vi "Teleop.vi"(10 "Match Info":T3={"Autonomous Elapsed Seconds"=0.0, "TeleOp Elapsed Seconds"=0.0, "Disabled Elapsed Seconds"=0.0, "Visited Autonomous"=FALSE, "Visited TeleOp"=FALSE, "Visited Disabled"=FALSE, "Autonomous Settings"={"Autonomous Style"=enum."Independent", "VI Refnum"=refnum}}, 11 "Call Context":T4) -> ()   [LabVIEW 2019]
doc: "This VI is called for each TeleOp packet received from the DS where the robot is not disabled. It is often used to read from the joysticks and update I/O or to update setpoints for timed control loops. It should complete and return within 20 milliseconds or it may miss DS packets."
uses:
  <vilib>/Rock Robotics/WPI/DriverStation/WPI_DriverStationDerivedRobotMode.ctl
  <vilib>/Rock Robotics/WPI/DriverStation/WPI_DriverStationMatch Info.ctl
  <vilib>/Rock Robotics/WPI/ThirdParty/Phoenix-LabVIEW/CANCoder/Controls/CTRE_Phoenix_CANcoder_StatusFrame.ctl
  <vilib>/Rock Robotics/WPI/ThirdParty/Phoenix-LabVIEW/CANCoder/Get/CTRE_Phoenix_CANcoder_GetSensorData.vi
panel:
  out "Sticky Faults":T1
  out "Faults":T1
  out "periodMs":u32
  in  "Period (ms)":u8=10
  in  "CANcoder Status Frame":T2=267264 items=["SensorData"=267264, "VbatAndFaults"=267328]
  out "Absolute Position":dbl
  out "Velocity":dbl(graph)
  out "Position":dbl(graph)
  in  "Set Status":bool
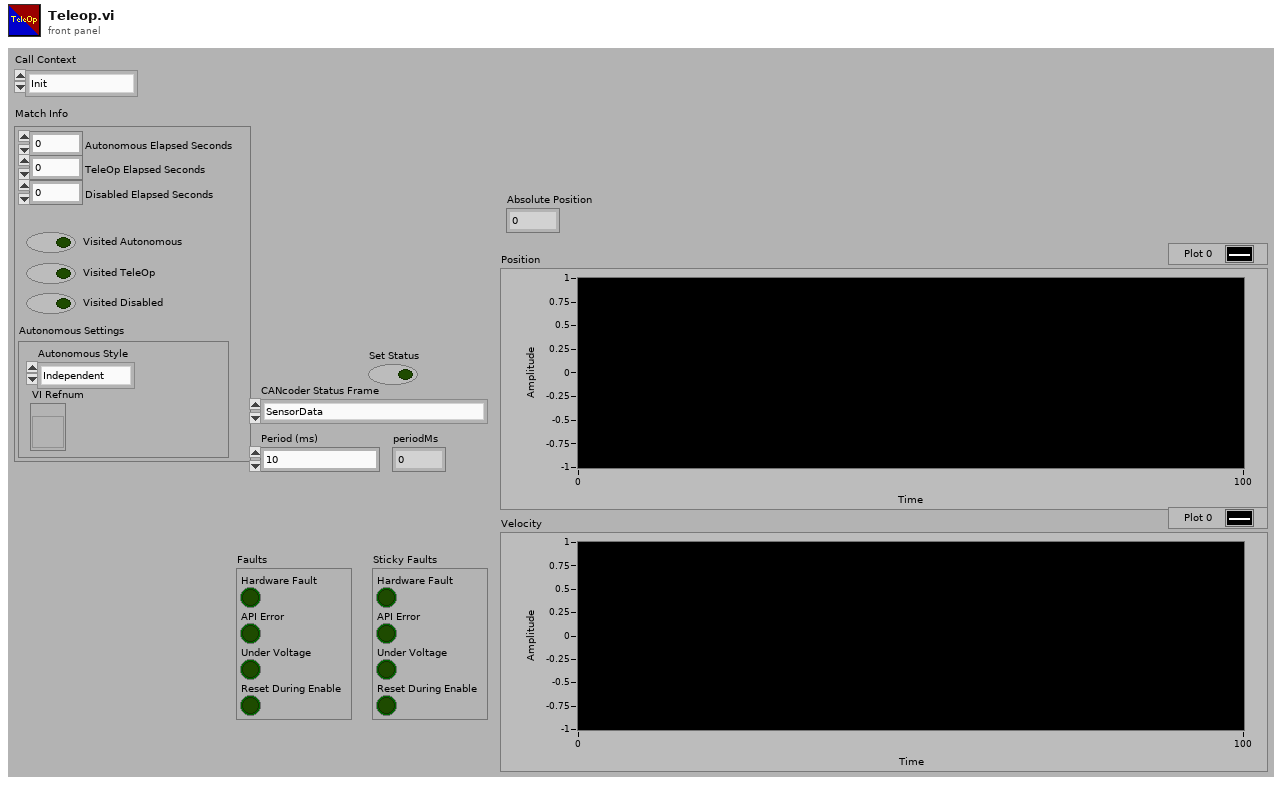
[diagram p1: front panel]
types:
  T1 = cluster{"Hardware Fault":bool, "API Error":bool, "Under Voltage":bool, "Reset During Enable":bool}
  T2 = typedef "CTRE_Phoenix_CANcoder_StatusFrame.ctl" = u32
  T3 = typedef "WPI_DriverStationMatch Info.ctl" = cluster{"Autonomous Elapsed Seconds":dbl, "TeleOp Elapsed Seconds":dbl, "Disabled Elapsed Seconds":dbl, "Visited Autonomous":bool, "Visited TeleOp":bool, "Visited Disabled":bool, "Autonomous Settings":cluster{"Autonomous Style":enum16{"Iterative", "Independent"}, "VI Refnum":refnum<vi>}}
  T4 = typedef "WPI_DriverStationDerivedRobotMode.ctl" = enum16{"Init", "Execute", "Stop"}
  T5 = typedef "CTRE_Phoenix_CANcoder_DeviceRef.ctl" = cluster{"DeviceStatus":errorcluster, "Device Number":u8, "Handle":u64, "UsageFrame":u32, "Library Path":path}
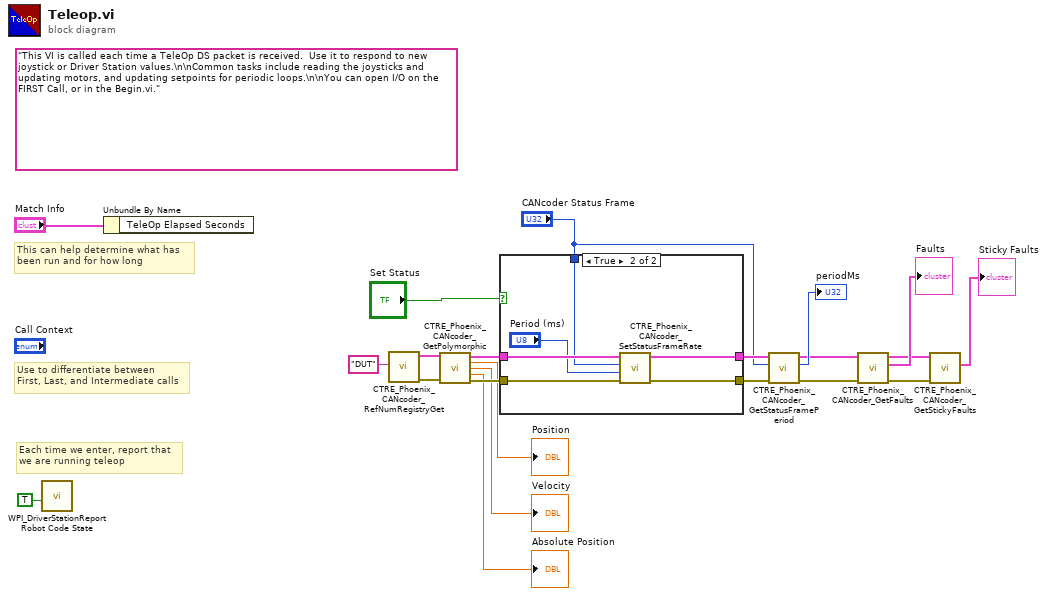
[diagram p0: block diagram]
diagram:
  (unwired) "This VI is called each time a TeleOp DS packet is received.  Use it to respond to new joystick or Driver Station values.\n\nCommon tasks include reading the joysticks and updating motors, and updating setpoints for periodic loops.\n\nYou can open I/O on the FIRST Call, or in the Begin.vi."
  # "Each time we enter, report that\nwe are running teleop"
  # "Use to differentiate between\nFirst, Last, and Intermediate calls"
  # "This can help determine what has\nbeen run and for how long"
  n1 = call <vilib>:"WPI_DriverStationReport Robot Code State.vi"("TeleOp"=TRUE ("Autonomous")) -> ()  [unwired: 10 in, 1 out]
  n2 = Unbundle By Name("Match Info") -> ()  [unwired: 1 out]
  n3 = call <vilib>:"CTRE_Phoenix_CANcoder_RefNumRegistryGet.vi"("refnum name"="DUT") -> ("error out"=w17:errorcluster, "CTRE_CANcoder_DeviceRef"=w18:T5)  [unwired: 9 in]
  n4 = call-poly <vilib>:"CTRE_Phoenix_CANcoder_GetPolymorphic.vi"("CTRE_CANcoder_DeviceRef"=w18, "error in"=w17) -> ("CTRE_CANcoder_DeviceRef"=w14:T5, "Position"=→"Position":dbl, "Velocity"=→"Velocity":dbl, "Absolute Position"=→"Absolute Position":dbl, "error out"=w15:errorcluster)  [unwired: 9 in]
  n5 = case shown="True" "Set Status" {
    tunnel: w15 -> [w22 w29]
    tunnel: w14 -> [w23 w28]
    tunnel: [w22 w26] -> w10
    tunnel: [w23 w25] -> w9
    tunnel: "CANcoder Status Frame" -> [_ w24]
    frame False {
    }
    frame True {
      n6 = call <vilib>:"CTRE_Phoenix_CANcoder_SetStatusFrameRate.vi"("error in (no error)"=w29, "Period (ms)"="Period (ms)", "CANcoder Status Frame"=w24, "CTRE_CANcoder_DeviceRef"=w28) -> ("error out"=w26:errorcluster, "CTRE_CANcoder_DeviceRef"=w25:T5)  [unwired: 6 in]
    }
  }
  n7 = call <vilib>:"CTRE_Phoenix_CANcoder_GetStatusFramePeriod.vi"("error in"=w10, "CANcoder Status Frame"="CANcoder Status Frame", "CTRE_CANcoder_DeviceRef"=w9) -> ("error out"=w6:errorcluster, "periodMs"=→"periodMs":u32, "CTRE_CANcoder_DeviceRef"=w5:T5)  [unwired: 6 in]
  n8 = call <vilib>:"CTRE_Phoenix_CANcoder_GetFaults.vi"("error in"=w6, "CTRE_CANcoder_DeviceRef"=w5) -> ("error out"=w2:errorcluster, "Faults"=→"Faults":T1, "CTRE_CANcoder_DeviceRef"=w3:T5)  [unwired: 7 in]
  n9 = call <vilib>:"CTRE_Phoenix_CANcoder_GetStickyFaults.vi"("error in"=w2, "CTRE_CANcoder_DeviceRef"=w3) -> ("Sticky Faults"=→"Sticky Faults":T1)  [unwired: 7 in, 2 out]
